vi "SCD - Trigger Sequence Generation.vi"(7 "Modulation Cycles\n per Wavelength":dbl=1.0 min=1.0 max=30.0 step=1.0, 8 "error in":errorcluster, 10 "FPS":dbl=10.0 min=1.0 max=30.0 step=1.0 format="%0.2p", 11 "LCVR Tuning Voltages":dbl[](array[numeric])=[2.507812176689576, 2.15366433871353, 1.9933549097130345, 1.7950985575543046, 1.7693912053041134] format="%.3g") -> (0 "error out":errorcluster, 1 "LCVR Relaxtion Time (ms)":dbl=200.0 format="%#_13g", 2 "AO Waveforms":waveform(dbl)[](array[waveform])=[{"t0"=timestamp(0 s since 1904-01-01), "dt"=0.000125, "Y"=array[4800 elements]}, {"t0"=timestamp(0 s since 1904-01-01), "dt"=0.000125, "Y"=array[4800 elements]}, {"t0"=timestamp(0 s since 1904-01-01), "dt"=0.000125, "Y"=array[4800 elements]}, {"t0"=timestamp(0 s since 1904-01-01), "dt"=0.000125, "Y"=array[4800 elements]}, {"t0"=timestamp(0 s since 1904-01-01), "dt"=0.000125, "Y"=array[4800 elements]}, {"t0"=timestamp(0 s since 1904-01-01), "dt"=0.000125, "Y"=array[4800 elements]}, {"t0"=timestamp(0 s since 1904-01-01), "dt"=0.000125, "Y"=array[4800 elements]}, {"t0"=timestamp(0 s since 1904-01-01), "dt"=0.000125, "Y"=array[4800 elements]}])   [LabVIEW 2014]
doc: "Nematic LC's require a modulation frequency of 2 kHz. If we sample each period with 4 samples, this means a sampling rate of 8000 samples per second = 125 microseconds per update\n\nThe default acquisition sequence is a \"Wavelength Tuning Relaxation Delay\" wherein no images are being acquired followed by a \"Wavelength Acquisition Interval\".\nThis is then repeated for 'n' wavelength intervals (typically 3 or 5).\n\nWe've decided (Matus and Scott) to just use external triggered mode acquisition for PDSS and SCD Instruments. In this mode, the rising edge of the trigger pulse initiates the camera exposure but the duration of the exposure is controlled by a pre-set camera clock. Therefore duty cycle for the trigger waveform generation is not important.\n\nThe delay before each wavelength interval is 2 sets of modulation cyles (2 x 133 ms = 266 ms)\n\nThis is because we're starting the modulation waveforms at the same time as we start the trigger delay and\nthe required time for 1 modulation cycle is 4 x 33.33 ms = 133 ms. In one modulation cycle, the LCVR's still\nwon't have completely tuned to the correct desired wavelength.\n\nIf we want to regain these 66 ms, we can delay the start of the modulation pulses to begin exactly at 200ms\n\n\nThis sequence depends on the exposure time being set to 33.3ms\n\nThe Goodrich Camera OPR Setting 22 produces an exposure (internally timed) of 31.994 ms.\nEach modulation state lasts 33.3 ms therefore the duty cycle of the trigger square is 31.994/33.3333 = 96%\n\nIt is important to have the phase be low enought so that there is not an articifial trigger pulse (this occurs at a phase of -15)\n\nWe've determined that a phase of -10 degrees and a duty cycle of 96% produce a camera exposure that lies entirely\nwithin a single modulation state."
uses:
  <vilib>/Waveform/WDTOps.llb/WDT Append Waveforms DBL.vi
  <vilib>/measure/NI_MABase.lvlib
panel:
  in  "LCVR Relaxtion (ms)":dbl=200.0 format="%#_13g"
  out "SCD AO Waveforms Graph":waveform(dbl)[](graph)=[{"t0"=timestamp(0 s since 1904-01-01), "dt"=0.000125, "Y"=array[4800 elements]}, {"t0"=timestamp(0 s since 1904-01-01), "dt"=0.000125, "Y"=array[4800 elements]}, {"t0"=timestamp(0 s since 1904-01-01), "dt"=0.000125, "Y"=array[4800 elements]}, {"t0"=timestamp(0 s since 1904-01-01), "dt"=0.000125, "Y"=array[4800 elements]}, {"t0"=timestamp(0 s since 1904-01-01), "dt"=0.000125, "Y"=array[4800 elements]}, {"t0"=timestamp(0 s since 1904-01-01), "dt"=0.000125, "Y"=array[4800 elements]}, {"t0"=timestamp(0 s since 1904-01-01), "dt"=0.000125, "Y"=array[4800 elements]}, {"t0"=timestamp(0 s since 1904-01-01), "dt"=0.000125, "Y"=array[4800 elements]}]
  # "User Adjustable Values are in this box"
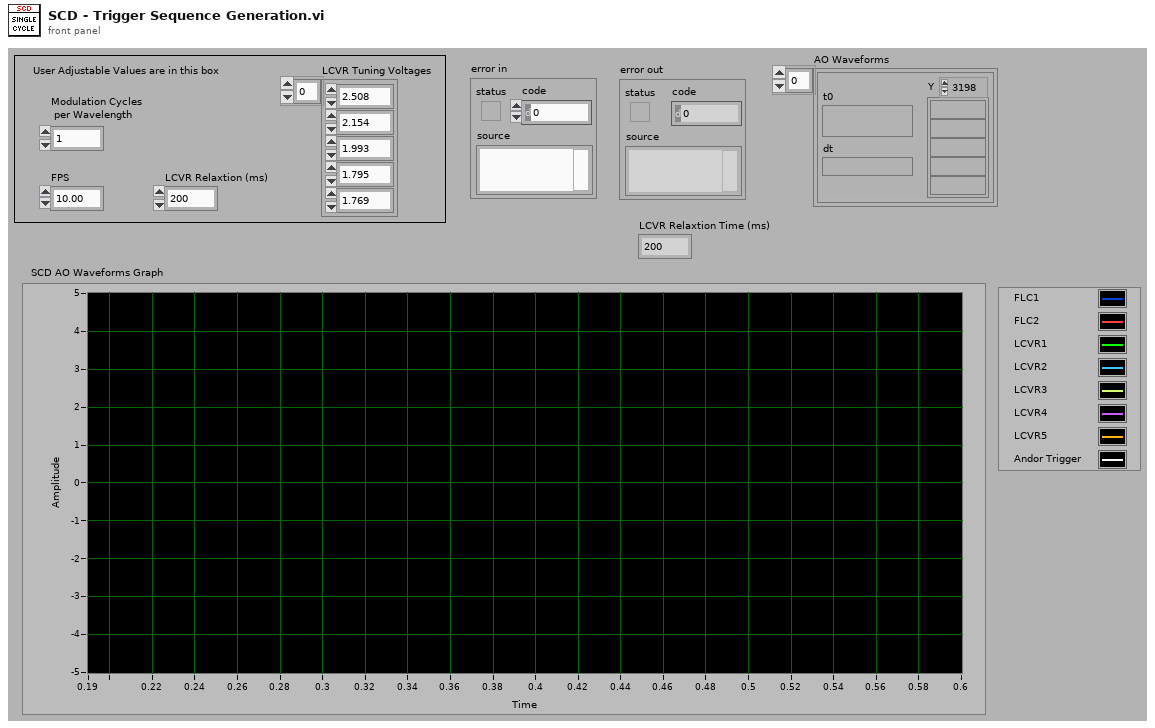
[diagram p1: front panel]
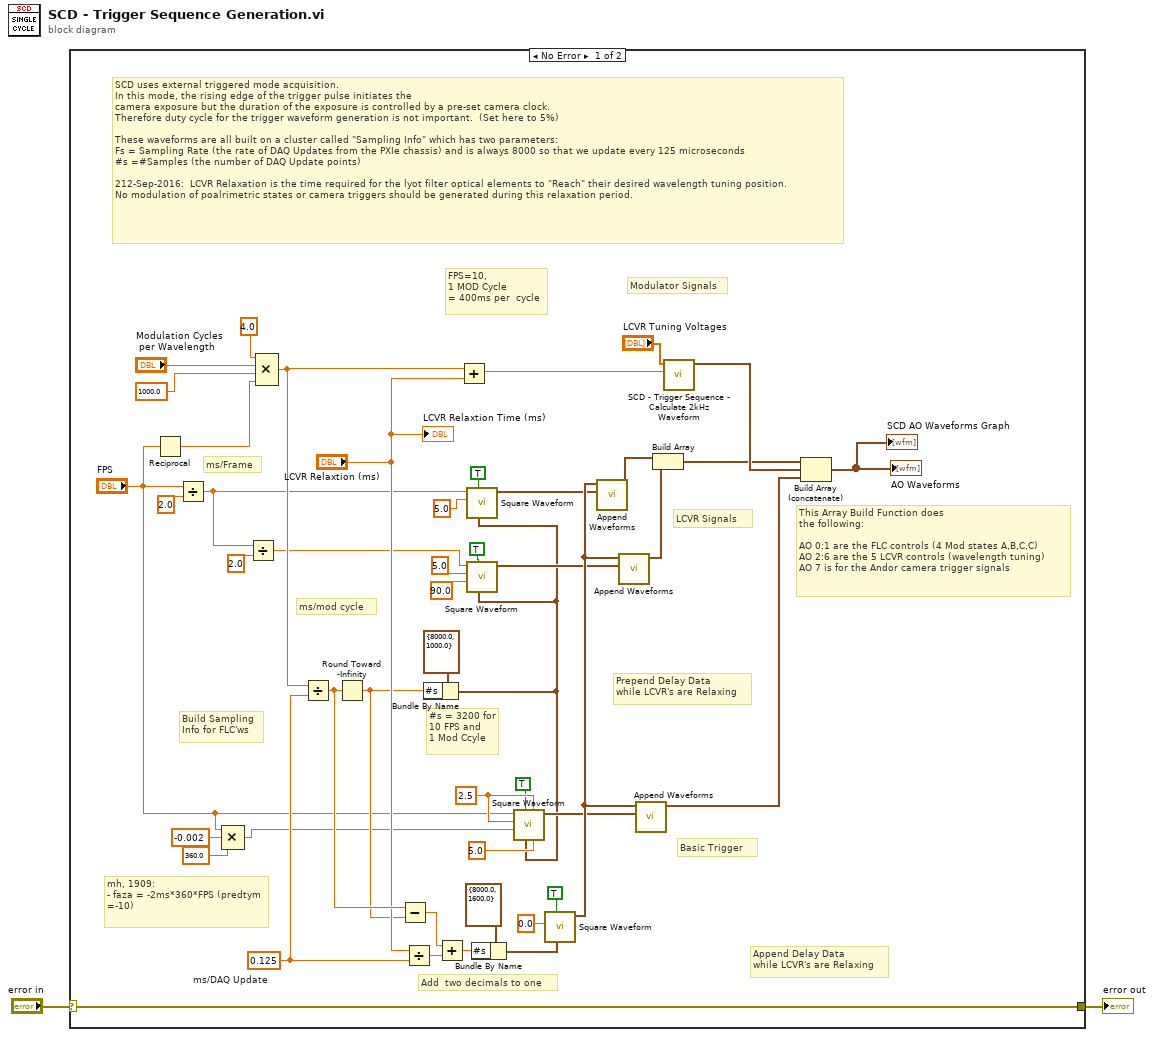
[diagram p0: block diagram]
diagram:
  n1 = case shown="No Error" "error in" {
    selector: "error in" -> [w49 w50]
    tunnel: [w49 w50] -> w1
    frame No Error {
      w26 = 2.5 ("Trigger Amp (V)")
      w19 = 0.125  # ms/DAQ Update
      # "Build Sampling\nInfo for FLC'ws"
      # "mh, 1909:\n- faza = -2ms*360*FPS (predtym =-10)"
      # "FPS=10,\n1 MOD Cycle\n= 400ms per  cycle"
      # "#s = 3200 for\n10 FPS and\n1 Mod Ccyle"
      # "This Array Build Function does\nthe following:\n\nAO 0:1 are the FLC controls (4 Mod states A,B,C,C)\nAO 2:6 are the 5 LCVR controls (wavelength tuning)\nAO 7 is for the Andor camera trigger signals"
      # "ms/mod cycle"
      # "ms/Frame"
      # "SCD uses external triggered mode acquisition.  \nIn this mode, the rising edge of the trigger pulse initiates the\ncamera exposure but the duration of the exposure is controlled by a pre-set camera clock.  \nTherefore duty cycle for the trigger waveform generation is not important.  (Set here to 5%)\n\nThese waveforms are all built on a cluster called \"Sampling Info\" which has two parameters:\nFs = Sampling Rate (the rate of DAQ Updates from the PXIe chassis) and is always 8000 so that we update every 125 microseconds\n#s =#Samples (the number of DAQ Update points)\n\n212-Sep-2016:  LCVR Relaxation is the time required for the lyot filter optical elements to \"Reach\" their desired wavelength tuning position.\nNo modulation of poalrimetric states or camera triggers should be generated during this relaxation period."
      # "Append Delay Data \nwhile LCVR's are Relaxing"
      # "Prepend Delay Data \nwhile LCVR's are Relaxing"
      # "Basic Trigger"
      # "Add  two decimals to one"
      # "LCVR Signals"
      # "Modulator Signals"
      n2 = Reciprocal(x="FPS") -> (1/x=w15:dbl)
      n3 = Divide(x="FPS", y=2.0) -> (x/y=w4:dbl)
      n4 = Compound Arithmetic op=MULTIPLY("FPS", -0.002 ("value"), 360.0 ("value")) -> (w6:dbl)
      n5 = Divide(x=w4, y=2.0) -> (x/y=w3:dbl)
      n6 = Compound Arithmetic op=MULTIPLY(4.0 ("Mod States Per Interval"), "Modulation Cycles\n per Wavelength", 1000.0 ("x"), w15) -> (w14:dbl)
      n7 = Divide(x=w14, y=w19) -> (x/y=w21:dbl)
      n8 = Round Toward -Infinity(1:w21) -> (0:w13:dbl)
      n9 = Subtract(x=w21, y=w13) -> (x-y=w36:dbl)
      n10 = Divide(x="LCVR Relaxtion (ms)", y=w19) -> (x/y=w38:dbl)
      n11 = Bundle By Name(cluster=cluster{"Fs":dbl, "#s":dbl} {"Fs"=8000.0, "#s"=1000.0} ("sampling info"), "#s"=w13) -> (w11:cluster{"Fs":dbl, "#s":dbl})
      n12 = Add(x=w36, y=w38) -> (x+y=w37:dbl)
      n13 = Add(x=w14, y="LCVR Relaxtion (ms)") -> (x+y=w29:dbl)
      n14 = call <vilib>:"Square Waveform.vi"("sampling info"=w11, "reset signal"=TRUE, "amplitude"=5.0 ("FLC #1 Amp (V)"), "frequency"=w4) -> ("signal out"=w33:waveform(dbl))  [unwired: 6 in, 1 out]
      n15 = call <vilib>:"Square Waveform.vi"("sampling info"=w11, "reset signal"=TRUE, "phase"=90.0 ("FLC2 Phase (deg)"), "amplitude"=5.0 ("FLC #2 Amp"), "frequency"=w3) -> ("signal out"=w31:waveform(dbl))  [unwired: 5 in, 1 out]
      n16 = Bundle By Name(cluster=cluster{"Fs":dbl, "#s":dbl} {"Fs"=8000.0, "#s"=1600.0} ("sampling info"), "#s"=w37) -> (w28:cluster{"Fs":dbl, "#s":dbl})
      n17 = call <vilib>:"Square Waveform.vi"("duty cycle (%)"=5.0, "offset"=w26, "sampling info"=w11, "reset signal"=TRUE, "phase"=w6, "amplitude"=w26, "frequency"="FPS") -> ("signal out"=w24:waveform(dbl))  [unwired: 3 in, 1 out]
      n18 = call <vilib>:"Square Waveform.vi"("sampling info"=w28, "reset signal"=TRUE, "amplitude"=0.0 ("Delay Voltage (no triggers)")) -> ("signal out"=w34:waveform(dbl))  [unwired: 7 in, 1 out]
      n19 = call-poly <vilib>:"Append Waveforms.vi"("waveform B"=w33, "waveform A"=w34) -> ("waveform out"=w32:waveform(dbl))  [unwired: 8 in, 1 out]
      n20 = call-poly <vilib>:"Append Waveforms.vi"("waveform B"=w31, "waveform A"=w34) -> ("waveform out"=w30:waveform(dbl))  [unwired: 8 in, 1 out]
      n21 = call-poly <vilib>:"Append Waveforms.vi"("waveform B"=w24, "waveform A"=w34) -> ("waveform out"=w27:waveform(dbl))  [unwired: 8 in, 1 out]
      n22 = Build Array(w32, w30) -> (w44:waveform(dbl)[])
      n23 = call "SCD - Trigger Sequence - Calculate 2kHz Waveform.vi"("Total Time (ms)"=w29, "Voltages"="LCVR Tuning Voltages") -> ("tuning waveforms"=w47:waveform(dbl)[])  [unwired: 8 in, 1 out]
      n24 = Build Array (concatenate)(w44, w47, w27) -> (→"AO Waveforms" →"SCD AO Waveforms Graph":waveform(dbl)[])
      "LCVR Relaxtion Time (ms)" <- "LCVR Relaxtion (ms)"
    }
    frame Error {
    }
  }
  "error out" <- w1
